vi "运维调试_质控单元.vi"() -> ()   [LabVIEW 2016, in "质控单元.lvlib"]
uses:
  <vilib>/Utility/miscctls.llb/LVPointTypeDef.ctl
  <vilib>/Plasmionique/MB Master/MB_Master_Serial/MB_Master_Serial.lvclass
  F:/Program Files/National Instruments/LabVIEW 2016/vi.lib/Plasmionique/MB Master/MB_Master/MB_Master.lvclass
  <vilib>/Plasmionique/MB Master/MB Master.lvlib
  <vilib>/ptbypt/NI_PtbyPt.lvlib
panel:
  out "COD液位传感器":bool
  out "氨氮总磷液位传感器":bool
  out "columns":string[](array[string])
  out "data":T1
  out "氨氮加标回收测完标志":bool
  out "COD加标回收测完标志":bool
  out "氨氮总磷加标回收测完标志":bool
  out "COD平行样测完标志":bool
  out "氨氮总磷平行样测完标志":bool
  out "输出簇 2":T2
  out "常规启动 2":bool
  out "直接启动 2":bool
  out "启动模块 2":cluster{"氨氮1":bool, "总磷1":bool, " COD1":bool}
  in  "停止测量":bool
  out "输出簇":T2
  in  "启动流程":T3(ring)
  out "启动模块":cluster{"氨氮1":bool, "总磷1":bool, " COD1":bool}
  out "直接启动":bool
  out "常规启动":bool
  out "COD传感器故障报警":bool
  in  "加标回收":bool
  in  "平行样测试":bool
  out "氨氮传感器故障报警":bool
  in  "CODMn停止":bool
  in  "CODMn排液":bool
  in  "CODMn调试":bool
  in  "总磷停止":bool
  in  "总磷排液":bool
  in  "总磷调试":bool
  out "CODMn加标回收率":dbl caption="加标回收率" format="%.2f"
  out "CODMn加标体积":dbl caption="加标体积" format="%.3f"
  out "CODMn母液浓度":dbl caption="加标母液浓度" format="%.2f"
  out "CODMn加标水杯定容体积":dbl caption="加标水杯定容体积" format="%.2f"
  out "CODMn加标后水样浓度":dbl caption="加标后水样浓度" format="%.2f"
  out "CODMn加标前水样浓度":dbl caption="加标前水样浓度" format="%.2f"
  out "CODMn检出限":dbl caption="检出限" format="%.2f"
  out "CODMn量程":dbl caption="量程" format="%.2f"
  out "CODMn状态":u16(ring) caption="状态" items=["待机", "润洗", "进样", "等待取液", "排液"]
  out "总磷加标回收率":dbl caption="加标回收率" format="%.2f"
  out "总磷加标体积":dbl caption="加标体积" format="%.3f"
  out "总磷母液浓度":dbl caption="加标母液浓度" format="%.3f"
  out "总磷加标水杯定容体积":dbl caption="加标水杯定容体积" format="%.2f"
  out "总磷加标后水样浓度":dbl caption="加标后水样浓度" format="%.3f"
  out "总磷加标前水样浓度":dbl caption="加标前水样浓度" format="%.3f"
  out "总磷检出限":dbl caption="检出限" format="%.3f"
  out "总磷量程":dbl caption="量程" format="%.2f"
  out "总磷状态":u16(ring) caption="状态" items=["待机", "润洗", "进样", "等待取液", "排液"]
  out "氨氮加标回收率":dbl caption="加标回收率" format="%.2f"
  out "氨氮加标体积":dbl caption="加标体积" format="%.3f"
  out "氨氮母液浓度":dbl caption="加标母液浓度" format="%.3f"
  out "氨氮加标水杯定容体积":dbl caption="加标水杯定容体积" format="%.2f"
  out "氨氮加标后水样浓度":dbl caption="加标后水样浓度" format="%.3f"
  out "氨氮加标前水样浓度":dbl caption="加标前水样浓度" format="%.3f"
  out "氨氮检出限":dbl caption="检出限" format="%.3f"
  out "氨氮量程":dbl caption="量程" format="%.2f"
  out "氨氮状态":u16(ring) caption="状态" items=["待机", "润洗", "进样", "等待取液", "排液"]
  in  "氨氮停止":bool
  in  "氨氮排液":bool
  in  "氨氮调试":bool
  # "CODMn质控参数"
  # "%"
  # "mL"
  # "mg/L"
  # "mL"
  # "mg/L"
  # "mg/L"
  # "mg/L"
  # "mg/L"
  # "总磷质控参数"
  # "%"
  # "mL"
  # "mg/L"
  # "mL"
  # "mg/L"
  # "mg/L"
  # "mg/L"
  # "mg/L"
  # "氨氮质控参数"
  # "%"
  # "mL"
  # "mg/L"
  # "mL"
  # "mg/L"
  # "mg/L"
  # "mg/L"
  # "mg/L"
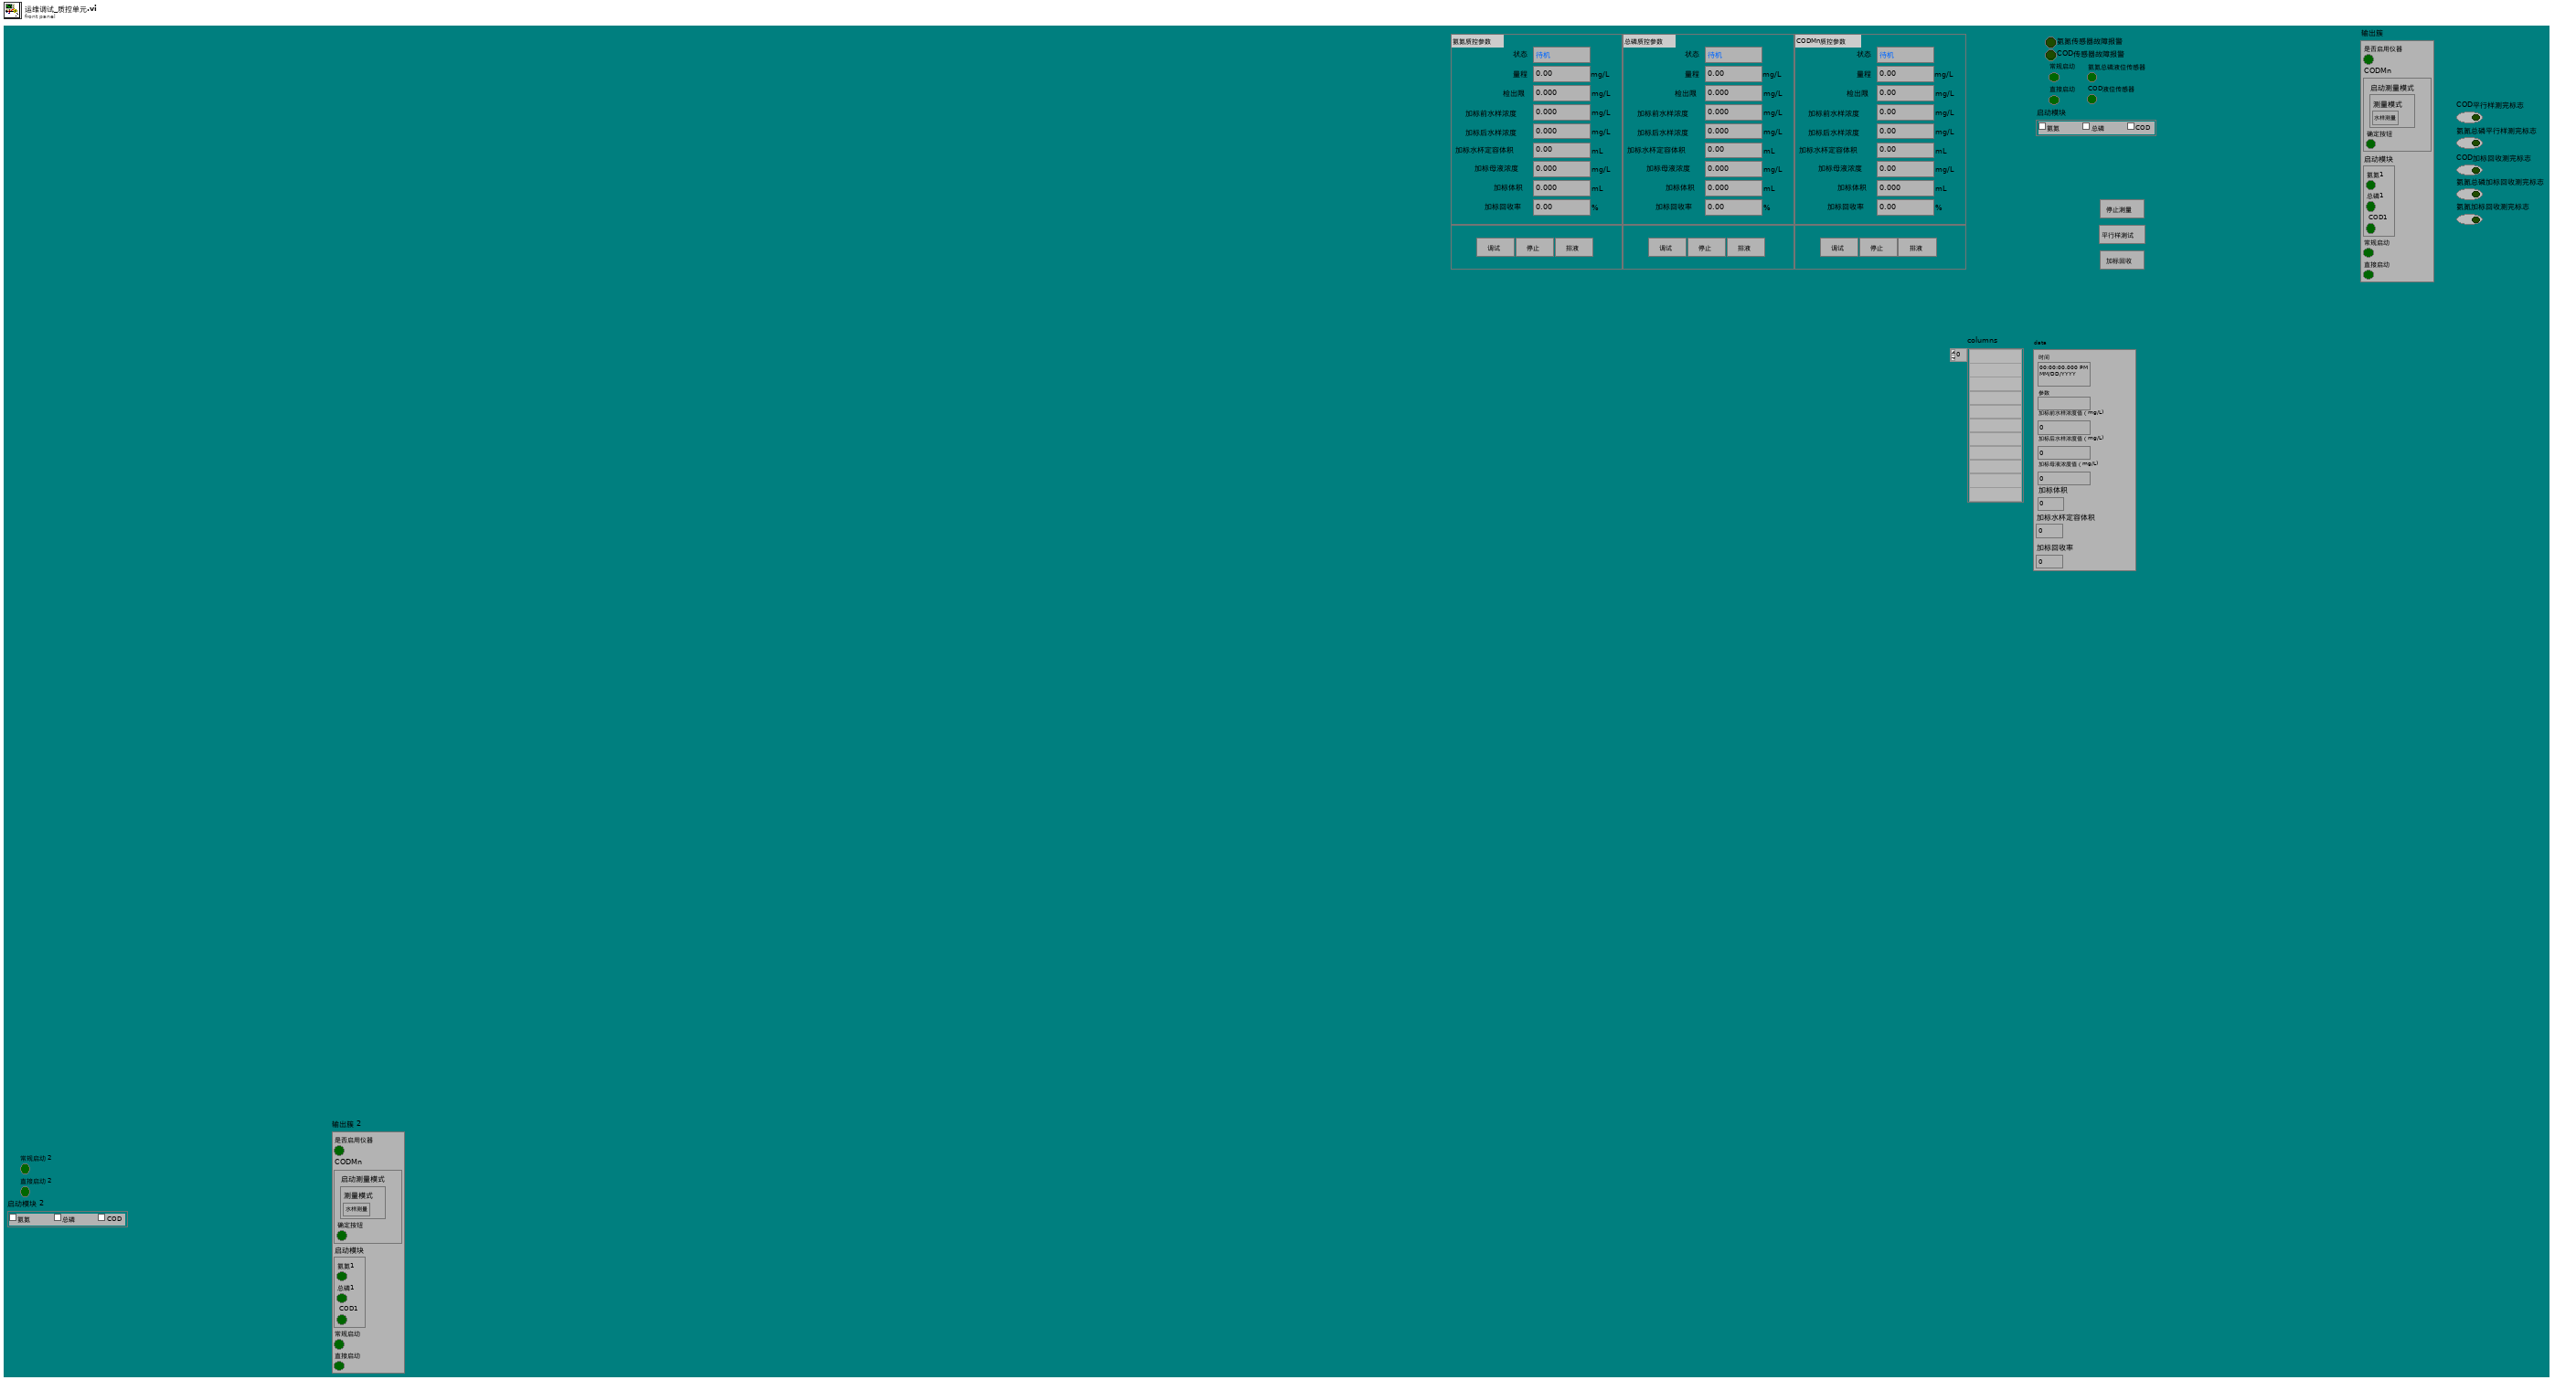
[diagram p1: front panel]
types:
  T1 = cluster{"时间":timestamp, "参数":string, "加标前水样浓度值（mg/L)":sgl, "加标后水样浓度值（mg/L)":sgl, "加标母液浓度值（mg/L)":sgl, "加标体积":dbl, "加标水杯定容体积":dbl, "加标回收率":dbl}
  T2 = cluster{"是否启用仪器":bool, "CODMn":cluster{"启动测量模式":cluster{"测量模式":enum16{"水样测量", "标样核查", "加标回收", "平行样", "校零", "校标"}}, "确定按钮":bool}, "启动模块":cluster{"氨氮1":bool, "总磷1":bool, " COD1":bool}, "常规启动":bool, "直接启动":bool}
  T3 = enum16{"初始化", "采配水", "测量水样", "加标", "取样测量", "测量结束"}
  T4 = cluster{"baud rate (bps)":u32, "stop bits":u16, "parity":u16, "flow control":u16, "timeout":u32, "retries":i32}
  T5 = typedef "LVPointTypeDef.ctl" = cluster{"Horizontal":i16, "Vertical":i16}
  T6 = cluster{"量程":dbl, "检出限":dbl, "加标前水样浓度":dbl, "加标后水样浓度":dbl, "加标水杯定容体积":dbl, "加标母液浓度":dbl, "加标体积":dbl, "加标回收率":dbl}
  T7 = cluster{"因子编码":u32, "单位":u16, "标样参考值":sgl, "水样数据时间":timestamp, "水样实测值":sgl, "水样数据标识":string, "标样数据时间":timestamp, "标样实测值":sgl, "标样数据标识":string, "空白数据时间":timestamp, "空白实测值":sgl, "空白数据标识":string, "零点核查数据时间":timestamp, "零点核查实测值":sgl, "零点核查数据标识":string, "跨度核查数据时间":timestamp, "跨度核查实测值":sgl, "跨度核查数据标识":string, "加标回收数据时间":timestamp, "加标回收实测值":sgl, "加标回收数据标识":string, "平行样数据时间":timestamp, "平行样实测值":sgl, "平行样数据标识":string}
  T8 = cluster{"时间":timestamp, "测量模式":string, "数据类型":string, "检测值":sgl, "单位":string, "数据标识":string, "因子编码":string, "标样参考值":sgl, "ORP-A":sgl, "ORP-B":sgl, "ORP-K":sgl, "COD滴定值":sgl, "高锰酸钾滴定数":sgl, "温度":sgl}
  T9 = enum8{"Enabled", "Disabled", "Disabled and Grayed Out"}
  T10 = cluster{"命令":string, cluster{"starting address":u16, "holding register value":u16}}
  T11 = enum32{"Bad", "Idle", "Run top level", "Running"}
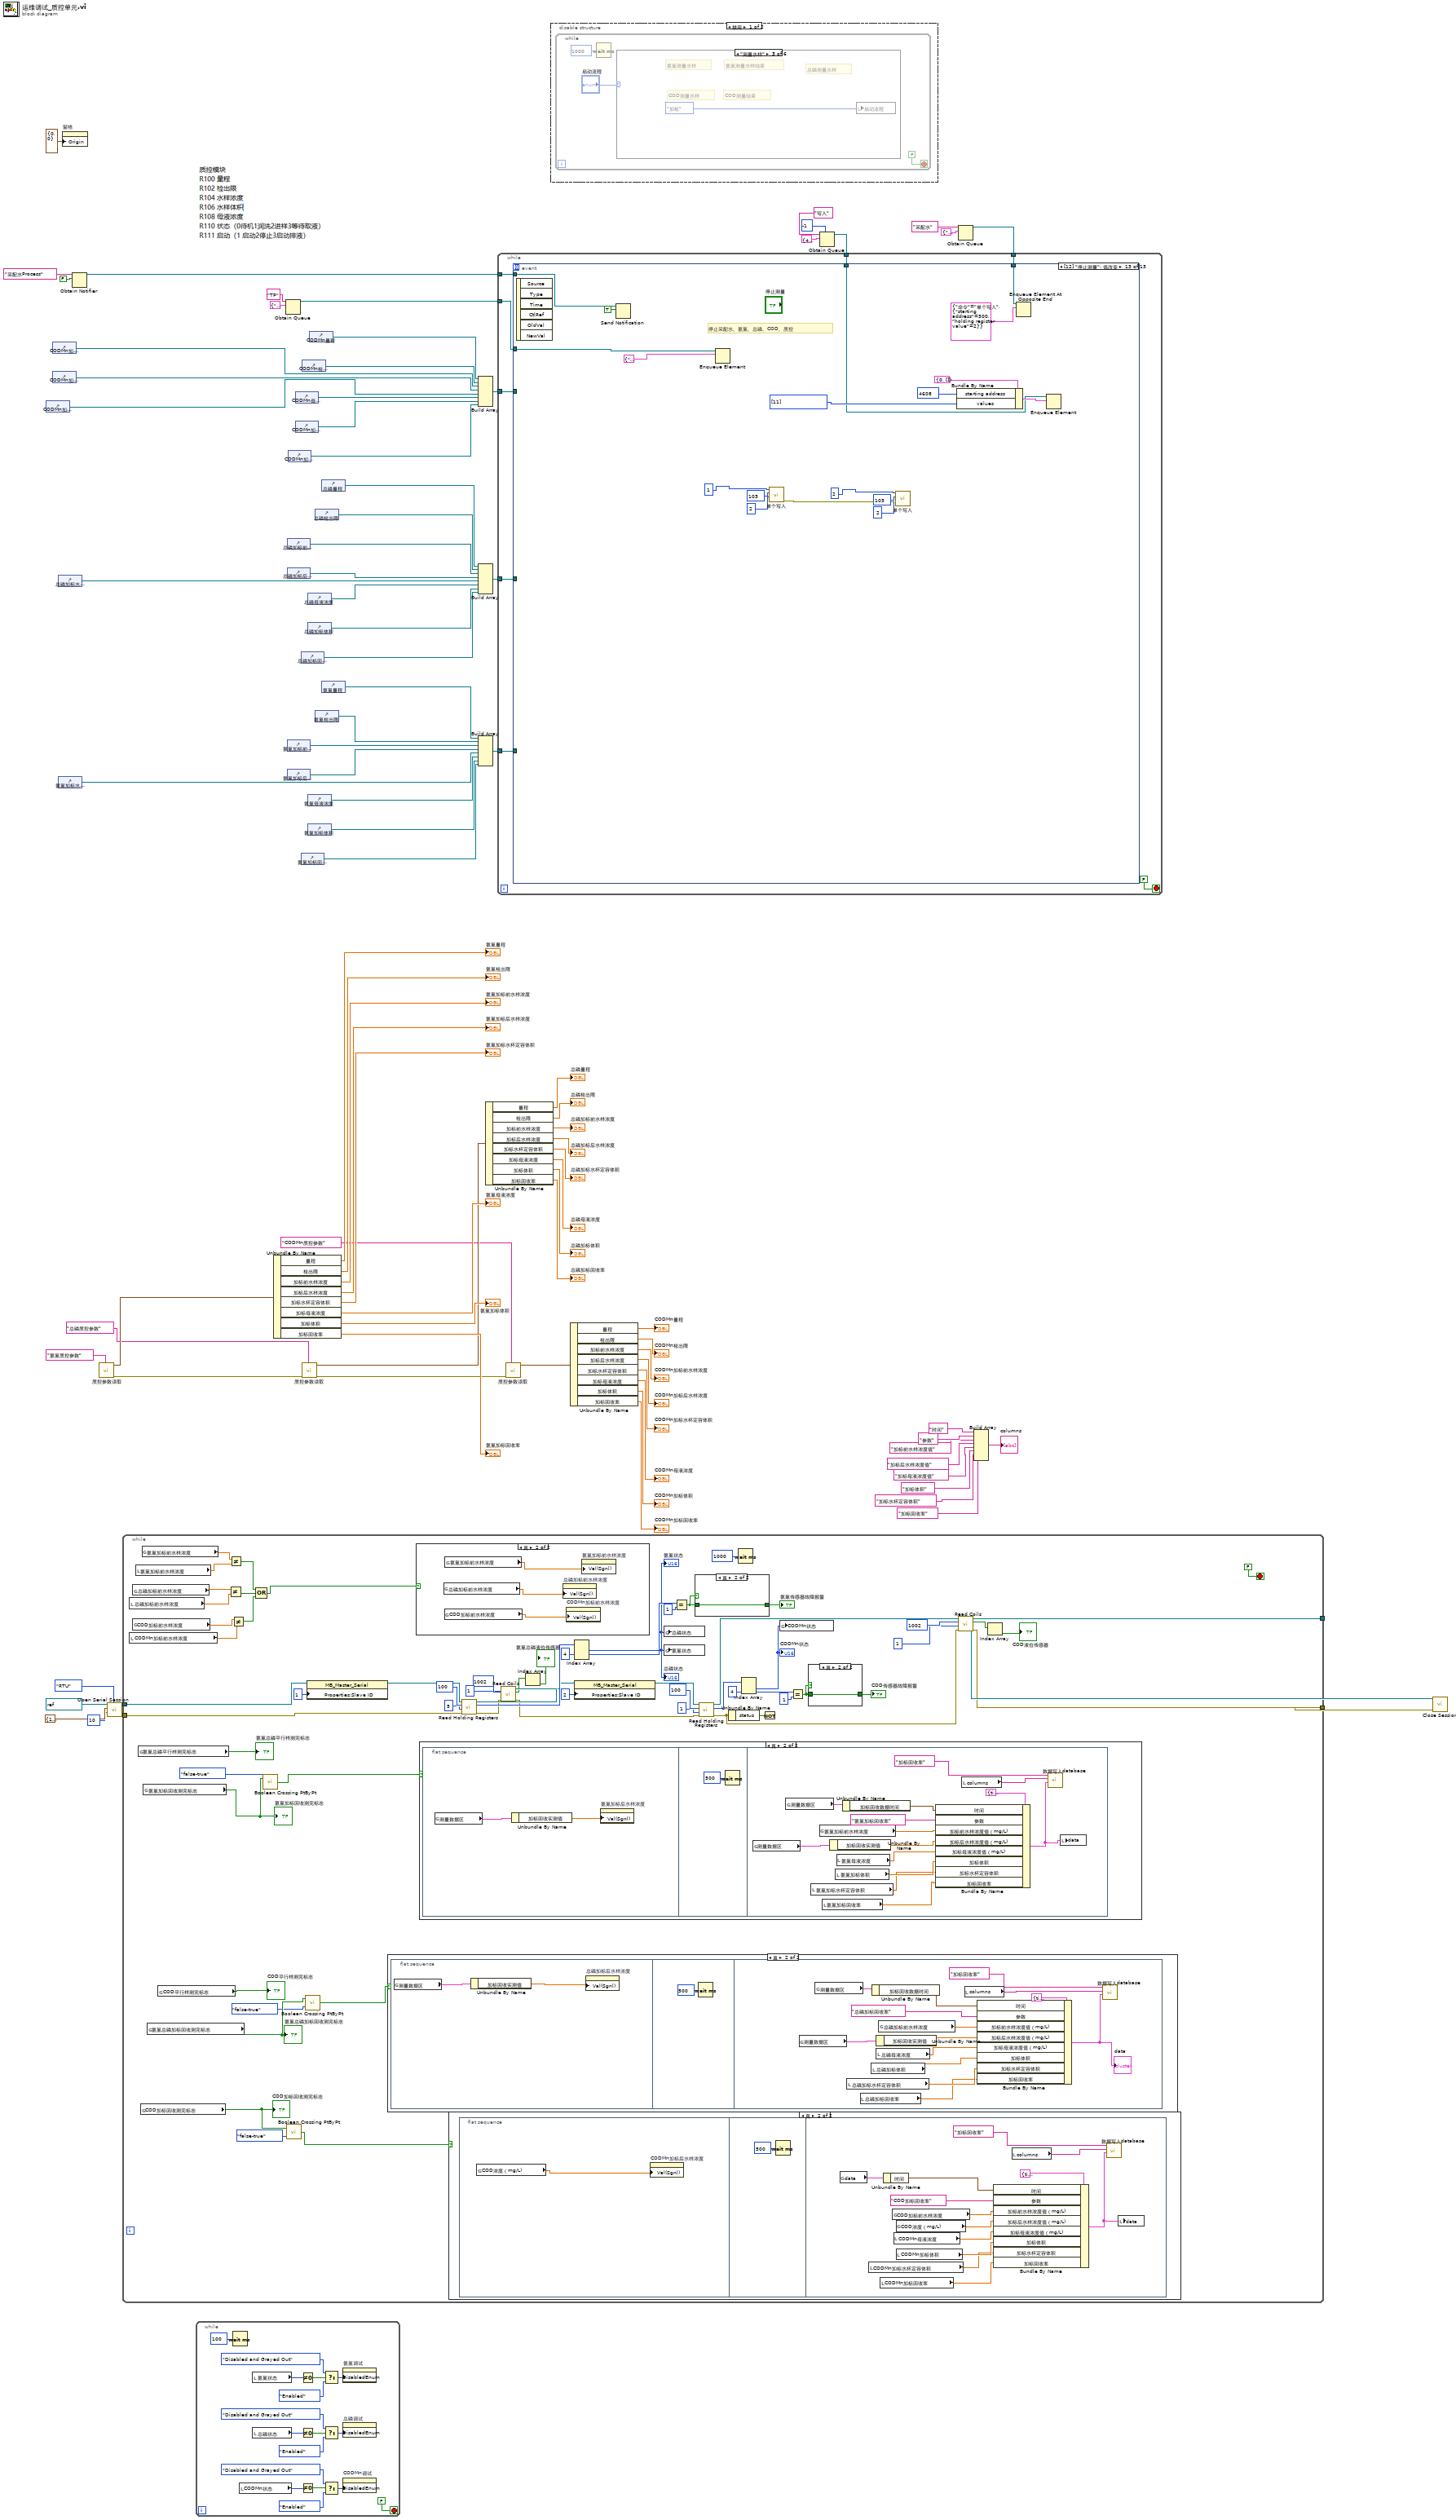
[diagram p0: block diagram]
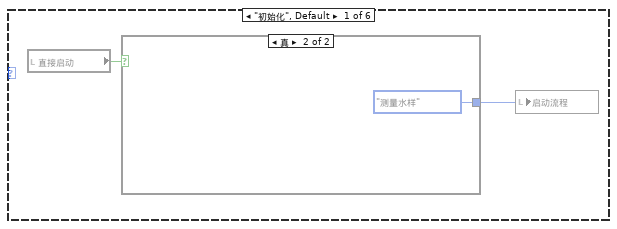
[diagram p2: hidden frame]
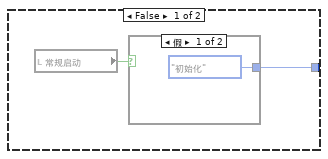
[diagram p3: hidden frame]
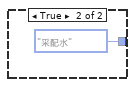
[diagram p4: hidden frame]
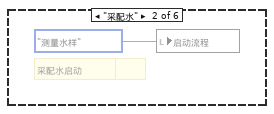
[diagram p5: hidden frame]
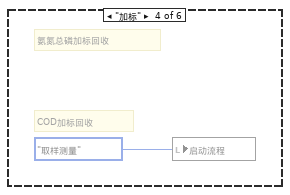
[diagram p6: hidden frame]
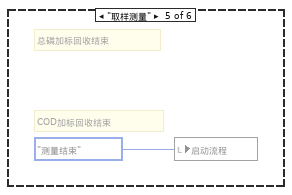
[diagram p7: hidden frame]
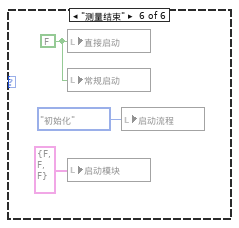
[diagram p8: hidden frame]
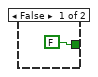
[diagram p14: hidden frame]
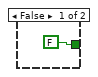
[diagram p15: hidden frame]
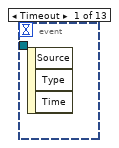
[diagram p16: hidden frame]
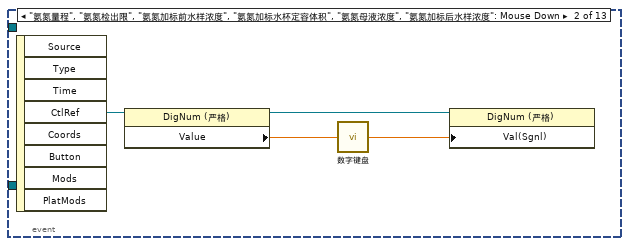
[diagram p17: hidden frame]
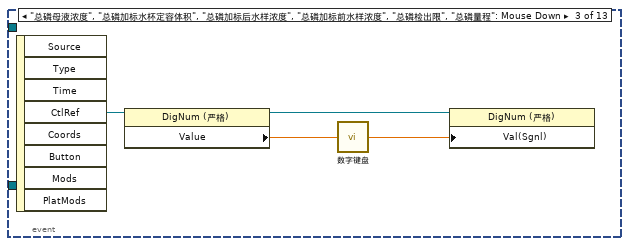
[diagram p18: hidden frame]
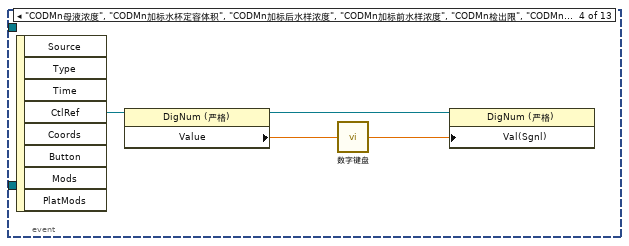
[diagram p19: hidden frame]
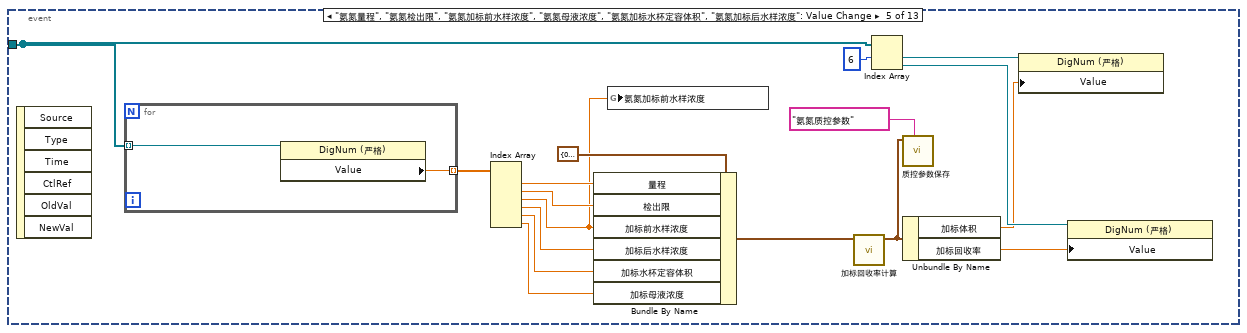
[diagram p20: hidden frame]
diagram:
  n1 = control-ref of="CODMn加标水杯定容体积"() -> (w35:refnum<vi>)
  n2 = control-ref of="CODMn加标前水样浓度"() -> (w37:refnum<vi>)
  n3 = control-ref of="CODMn加标后水样浓度"() -> (w36:refnum<vi>)
  n4 = control-ref of="总磷加标水杯定容体积"() -> (w44:refnum<vi>)
  n5 = control-ref of="氨氮加标水杯定容体积"() -> (w86:refnum<vi>)
  n6 = property on="窗格" class="Pane"("Origin"=T5 {"Horizontal"=0, "Vertical"=0} ("原点")) -> ()  [unwired: 2 in, 2 out]
  n7 = Obtain Notifier(name (unnamed)="采配水Process" ("名称（未命名）"), notification data type=FALSE) -> (notifier out=w20:refnum<notifier>)  [unwired: 2 in, 2 out]
  n8 = call "质控参数读取.vi"("section"="氨氮质控参数") -> ("error out"=w60:errorcluster, "参数"=w79:T6)  [unwired: 9 in]
  n9 = call <vilib>:"Open Serial Session.vi"("Mode (RTU)"=enum16{"RTU", "ASCII"}."RTU", "Slave ID"=u8 10, "Serial Config"=T4 {"baud rate (bps)"=115200, "stop bits"=10, "parity"=0, "flow control"=0, "timeout"=100, "retries"=1}, "VISA Resource"=refnum<visa-resource-name> "COM6") -> ("Error out"=w29:errorcluster, "MB_Serial session"=w30:refnum<class "MB_Master_Serial.lvclass">)  [unwired: 6 in]
  n10 = while {
    tunnel: w30 -> [w152]
    tunnel: w29 -> [w151]
    tunnel: [w97] -> w28
    tunnel: [w91] -> w27
    stop <- FALSE stop-if-true
    n11 = local read "总磷加标前水样浓度"() -> (w122:dbl)
    n12 = local read "CODMn加标前水样浓度"() -> (w120:dbl)
    n13 = global read "水样浓度全局.vi" "COD加标前水样浓度"() -> (w121:dbl)
    n14 = global read "水样浓度全局.vi" "总磷加标前水样浓度"() -> (w123:dbl)
    n15 = local read "氨氮加标前水样浓度"() -> (w124:dbl)
    n16 = global read "质控测完标志全局 1.vi" "氨氮总磷平行样测完标志"() -> (→"氨氮总磷平行样测完标志":bool)
    n17 = global read "质控测完标志全局 1.vi" "COD加标回收测完标志"() -> (w107:bool)
    "COD加标回收测完标志" <- w107
    n18 = global read "水样浓度全局.vi" "氨氮加标前水样浓度"() -> (w125:dbl)
    n19 = global read "质控测完标志全局 1.vi" "氨氮加标回收测完标志"() -> (w113:bool)
    "氨氮加标回收测完标志" <- w113
    n20 = global read "质控测完标志全局 1.vi" "氨氮总磷加标回收测完标志"() -> (w110:bool)
    "氨氮总磷加标回收测完标志" <- w110
    n21 = global read "质控测完标志全局 1.vi" "COD平行样测完标志"() -> (→"COD平行样测完标志":bool)
    n22 = Not Equal?(x=w123, y=w122) -> (x != y?=w117:bool)
    n23 = Not Equal?(x=w125, y=w124) -> (x != y?=w119:bool)
    n24 = Not Equal?(x=w121, y=w120) -> (x != y?=w116:bool)
    n25 = Compound Arithmetic op=OR ("复合运算")(w119, w117, w116) -> (w118:bool)
    n26 = call <vilib>:"Boolean Crossing PtByPt.vi"("direction"=enum16{"either", "false-true", "true-false"}."false-true", "input"=w113) -> ("crossing"=w112:bool)  [unwired: 1 in]
    n27 = call <vilib>:"Boolean Crossing PtByPt.vi"("direction"=enum16{"either", "false-true", "true-false"}."false-true", "input"=w107) -> ("crossing"=w105:bool)  [unwired: 1 in]
    n28 = call <vilib>:"Boolean Crossing PtByPt.vi"("direction"=enum16{"either", "false-true", "true-false"}."false-true", "input"=w110) -> ("crossing"=w108:bool)  [unwired: 1 in]
    n29 = property class="MB_Master_Serial"(reference=w152, "Properties:Slave ID"=u8 1 ("Slave ID")) -> (reference out=w139:refnum<class "MB_Master_Serial.lvclass">)  [unwired: 1 in, 1 out]
    n30 = case shown="真" w108 {
      frame False {
      }
      frame True {
        n31 = flat-sequence {
          frame #0 {
            n32 = global read "VAR总磷氨氮全局变量.vi" "测量数据区"() -> (w171:T7)
            n33 = Unbundle By Name(w171) -> ("加标回收实测值"=w170:sgl)
            n34 = property on="总磷加标后水样浓度" class="DigNum (严格)"("Val(Sgnl)"=w170) -> ()  [unwired: 2 in, 2 out]
          }
          frame #1 {
            n35 = Wait (ms)(milliseconds to wait=u32 500 ("等待时间（毫秒）")) -> ()  [unwired: 1 out]
          }
          frame #2 {
            n36 = global read "VAR总磷氨氮全局变量.vi" "测量数据区"() -> (w181:T7)
            n37 = global read "VAR总磷氨氮全局变量.vi" "测量数据区"() -> (w174:T7)
            n38 = local read "总磷加标水杯定容体积"() -> (w177:dbl)
            n39 = local read "总磷加标回收率"() -> (w176:dbl)
            n40 = local read "总磷加标体积"() -> (w178:dbl)
            n41 = Unbundle By Name(w174) -> ("加标回收数据时间"=w173:timestamp)
            n42 = Unbundle By Name(w181) -> ("加标回收实测值"=w180:sgl)
            n43 = local read "总磷母液浓度"() -> (w179:dbl)
            n44 = global read "水样浓度全局.vi" "总磷加标前水样浓度"() -> (w182:dbl)
            n45 = local read "columns"() -> (w185:string[])
            n46 = Bundle By Name(cluster=T1 {"时间"=timestamp(0 s since 1904-01-01), "参数"="", "加标前水样浓度值（mg/L)"=0.0, "加标后水样浓度值（mg/L)"=0.0, "加标母液浓度值（mg/L)"=0.0, "加标体积"=0.0, "加标水杯定容体积"=0.0, "加标回收率"=0.0} ("data"), "时间"=w173, "参数"="总磷加标回收率" ("table"), "加标前水样浓度值（mg/L)"=w182, "加标后水样浓度值（mg/L)"=w180, "加标母液浓度值（mg/L)"=w179, "加标体积"=w178, "加标水杯定容体积"=w177, "加标回收率"=w176) -> (w175:T1)
            "data" <- w175
            n47 = call "数据写入database.vi"("data"=w175, "columns"=w185, "table"="加标回收率") -> ()  [unwired: 9 in]
          }
        }
      }
    }
    n48 = case shown="真" w118 {
      frame False {
      }
      frame True {
        n49 = global read "水样浓度全局.vi" "总磷加标前水样浓度"() -> (w205:dbl)
        n50 = global read "水样浓度全局.vi" "COD加标前水样浓度"() -> (w204:dbl)
        n51 = global read "水样浓度全局.vi" "氨氮加标前水样浓度"() -> (w206:dbl)
        n52 = property on="总磷加标前水样浓度" class="DigNum (严格)"("Val(Sgnl)"=w205) -> ()  [unwired: 2 in, 2 out]
        n53 = property on="CODMn加标前水样浓度" class="DigNum (严格)"("Val(Sgnl)"=w204) -> ()  [unwired: 2 in, 2 out]
        n54 = property on="氨氮加标前水样浓度" class="DigNum (严格)"("Val(Sgnl)"=w206) -> ()  [unwired: 2 in, 2 out]
      }
    }
    n55 = case shown="真" w112 {
      frame False {
      }
      frame True {
        n56 = flat-sequence {
          frame #0 {
            n57 = global read "VAR总磷氨氮全局变量.vi" "测量数据区"() -> (w188:T7)
            n58 = Unbundle By Name(w188) -> ("加标回收实测值"=w187:sgl)
            n59 = property on="氨氮加标后水样浓度" class="DigNum (严格)"("Val(Sgnl)"=w187) -> ()  [unwired: 2 in, 2 out]
          }
          frame #1 {
            n60 = Wait (ms)(milliseconds to wait=u32 500 ("等待时间（毫秒）")) -> ()  [unwired: 1 out]
          }
          frame #2 {
            n61 = global read "VAR总磷氨氮全局变量.vi" "测量数据区"() -> (w196:T7)
            n62 = global read "VAR总磷氨氮全局变量.vi" "测量数据区"() -> (w200:T7)
            n63 = local read "氨氮加标水杯定容体积"() -> (w192:dbl)
            n64 = global read "水样浓度全局.vi" "氨氮加标前水样浓度"() -> (w197:dbl)
            n65 = local read "氨氮加标回收率"() -> (w191:dbl)
            n66 = Unbundle By Name(w196) -> ("加标回收实测值"=w195:sgl)
            n67 = local read "氨氮加标体积"() -> (w193:dbl)
            n68 = local read "氨氮母液浓度"() -> (w194:dbl)
            n69 = Unbundle By Name(w200) -> ("加标回收数据时间"=w199:timestamp)
            n70 = Bundle By Name(cluster=T1 {"时间"=timestamp(0 s since 1904-01-01), "参数"="", "加标前水样浓度值（mg/L)"=0.0, "加标后水样浓度值（mg/L)"=0.0, "加标母液浓度值（mg/L)"=0.0, "加标体积"=0.0, "加标水杯定容体积"=0.0, "加标回收率"=0.0} ("data"), "时间"=w199, "参数"="氨氮加标回收率" ("table"), "加标前水样浓度值（mg/L)"=w197, "加标后水样浓度值（mg/L)"=w195, "加标母液浓度值（mg/L)"=w194, "加标体积"=w193, "加标水杯定容体积"=w192, "加标回收率"=w191) -> (w190:T1)
            n71 = local read "columns"() -> (w202:string[])
            n72 = call "数据写入database.vi"("data"=w190, "columns"=w202, "table"="加标回收率") -> ()  [unwired: 9 in]
            n73 = local write "data"(w190) -> ()
          }
        }
      }
    }
    n74 = case shown="真" w105 {
      frame False {
      }
      frame True {
        n75 = flat-sequence {
          frame #0 {
            n76 = global read "COD浓度全局变量.vi" "COD浓度（mg/L)"() -> (w155:dbl)
            n77 = property on="CODMn加标后水样浓度" class="DigNum (严格)"("Val(Sgnl)"=w155) -> ()  [unwired: 2 in, 2 out]
          }
          frame #1 {
            n78 = Wait (ms)(milliseconds to wait=u32 500 ("等待时间（毫秒）")) -> ()  [unwired: 1 out]
          }
          frame #2 {
            n79 = global read "COD读取DATA全局.vi" "data"() -> (w165:T8)
            n80 = local read "CODMn加标水杯定容体积"() -> (w159:dbl)
            n81 = local read "CODMn加标回收率"() -> (w158:dbl)
            n82 = Unbundle By Name(w165) -> ("时间"=w164:timestamp)
            n83 = global read "水样浓度全局.vi" "COD加标前水样浓度"() -> (w163:dbl)
            n84 = local read "CODMn母液浓度"() -> (w161:dbl)
            n85 = global read "COD浓度全局变量.vi" "COD浓度（mg/L)"() -> (w162:dbl)
            n86 = local read "CODMn加标体积"() -> (w160:dbl)
            n87 = Bundle By Name(cluster=T1 {"时间"=timestamp(0 s since 1904-01-01), "参数"="", "加标前水样浓度值（mg/L)"=0.0, "加标后水样浓度值（mg/L)"=0.0, "加标母液浓度值（mg/L)"=0.0, "加标体积"=0.0, "加标水杯定容体积"=0.0, "加标回收率"=0.0} ("data"), "时间"=w164, "参数"="COD加标回收率" ("table"), "加标前水样浓度值（mg/L)"=w163, "加标后水样浓度值（mg/L)"=w162, "加标母液浓度值（mg/L)"=w161, "加标体积"=w160, "加标水杯定容体积"=w159, "加标回收率"=w158) -> (w157:T1)
            n88 = local read "columns"() -> (w168:string[])
            n89 = call "数据写入database.vi"("data"=w157, "columns"=w168, "table"="加标回收率") -> ()  [unwired: 9 in]
            n90 = local write "data"(w157) -> ()
          }
        }
      }
    }
    n91 = call <vilib>:"Read Holding Registers.vi"("error in (no error)"=w151, "quantity"=u16 5, "starting address"=u16 100, "MB session in"=w139) -> ("error out"=w100:errorcluster, "Registers"=w147:u16[], "MB session out"=w142:refnum<class "MB_Master_Serial.lvclass">)  [unwired: 5 in]
    n92 = call <vilib>:"Read Coils.vi"("error in (no error)"=w100, "quantity"=u16 1, "starting address"=u16 1002, "MB session in"=w142) -> ("error out"=w99:errorcluster, "Coils"=w101:bool[], "MB session out"=w104:refnum<class "MB_Master_Serial.lvclass">)  [unwired: 5 in]
    n93 = Index Array(array=w101) -> (element=→"氨氮总磷液位传感器":bool)  [unwired: 1 in]
    n94 = Index Array(array=w147, index #2=4 ("索引")) -> (element #1=w127:u16, element #2=w136:u16)  [unwired: 2 in, 1 out]
    "氨氮状态" <- w127
    "总磷状态" <- w127
    n95 = property class="MB_Master_Serial"(reference=w104, "Properties:Slave ID"=u8 2 ("Slave ID")) -> (reference out=w141:refnum<class "MB_Master_Serial.lvclass">)  [unwired: 1 in, 1 out]
    n96 = global write "氨氮加标回收状态全局变量.vi" "总磷状态"(w127) -> ()
    n97 = global write "氨氮加标回收状态全局变量.vi" "氨氮状态"(w127) -> ()
    n98 = Equal?(x=w136, y=u16 1) -> (x = y?=w133:bool)
    n99 = case shown="真" w133 {
      tunnel: w133 -> [_ w210]
      tunnel: [FALSE w210] -> w134
      frame False {
      }
      frame True {
      }
    }
    "氨氮传感器故障报警" <- w134
    n100 = call <vilib>:"Read Holding Registers.vi"("error in (no error)"=w99, "quantity"=u16 1, "starting address"=u16 100, "MB session in"=w141) -> ("error out"=w92:errorcluster, "Registers"=w146:u16[], "MB session out"=w150:refnum<class "MB_Master_Serial.lvclass">)  [unwired: 5 in]
    n101 = Unbundle By Name(w92) -> ("status"=w143:bool)
    n102 = Wait (ms)(milliseconds to wait=u32 1000 ("等待时间（毫秒）")) -> ()  [unwired: 1 out]
    n103 = Index Array(array=w146, index #2=4 ("索引")) -> (element #1=w126:u16, element #2=w130:u16)  [unwired: 1 in]
    "CODMn状态" <- w126
    n104 = Not(x=w143) -> ()  [unwired: 1 out]
    n105 = global write "氨氮加标回收状态全局变量.vi" "CODMn状态"(w126) -> ()
    n106 = Equal?(x=w130, y=u16 1) -> (x = y?=w128:bool)
    n107 = case shown="真" w128 {
      tunnel: w128 -> [_ w208]
      tunnel: [FALSE w208] -> w129
      frame False {
      }
      frame True {
      }
    }
    "COD传感器故障报警" <- w129
    n108 = call <vilib>:"Read Coils.vi"("error in (no error)"=w92, "quantity"=u16 1, "starting address"=u16 1002, "MB session in"=w150) -> ("error out"=w91:errorcluster, "Coils"=w94:bool[], "MB session out"=w97:refnum<class "MB_Master_Serial.lvclass">)  [unwired: 5 in]
    n109 = Index Array(array=w94) -> (element=→"COD液位传感器":bool)  [unwired: 1 in]
  }
  n110 = while {
    stop <- FALSE stop-if-true
    n111 = Wait (ms)(milliseconds to wait=u32 100 ("等待时间（毫秒）")) -> ()  [unwired: 1 out]
    n112 = local read "CODMn状态"() -> (w212:u16)
    n113 = local read "氨氮状态"() -> (w226:u16)
    n114 = local read "总磷状态"() -> (w217:u16)
    n115 = Not Equal To 0?(x=w226) -> (x != 0?=w225:bool)
    n116 = Not Equal To 0?(x=w217) -> (x != 0?=w219:bool)
    n117 = Not Equal To 0?(x=w212) -> (x != 0?=w216:bool)
    n118 = Select(t=T9."Disabled and Grayed Out" ("禁用"), s=w225, f=T9."Enabled") -> (s? t:f=w222:T9)
    n119 = Select(t=T9."Disabled and Grayed Out" ("禁用"), s=w219, f=T9."Enabled") -> (s? t:f=w218:T9)
    n120 = Select(t=T9."Disabled and Grayed Out" ("禁用"), s=w216, f=T9."Enabled") -> (s? t:f=w213:T9)
    n121 = property on="氨氮调试" class="Bool"("DisabledEnum"=w222) -> ()  [unwired: 2 in, 2 out]
    n122 = property on="总磷调试" class="Bool"("DisabledEnum"=w218) -> ()  [unwired: 2 in, 2 out]
    n123 = property on="CODMn调试" class="Bool"("DisabledEnum"=w213) -> ()  [unwired: 2 in, 2 out]
  }
  n124 = Unbundle By Name(w79) -> ("量程"=→"氨氮量程":dbl, "检出限"=→"氨氮检出限":dbl, "加标前水样浓度"=→"氨氮加标前水样浓度":dbl, "加标后水样浓度"=→"氨氮加标后水样浓度":dbl, "加标水杯定容体积"=→"氨氮加标水杯定容体积":dbl, "加标母液浓度"=→"氨氮母液浓度":dbl, "加标体积"=→"氨氮加标体积":dbl, "加标回收率"=→"氨氮加标回收率":dbl)
  n125 = Obtain Queue(name (unnamed)="TP" ("名称（未命名）"), element data type=cluster{"命令":string, "data":variant} {"命令"="", "data"=variant}) -> (queue out=w8:refnum<queue>)  [unwired: 3 in, 2 out]
  n126 = control-ref of="总磷加标前水样浓度"() -> (w46:refnum<vi>)
  n127 = control-ref of="总磷加标后水样浓度"() -> (w45:refnum<vi>)
  n128 = control-ref of="氨氮加标前水样浓度"() -> (w87:refnum<vi>)
  n129 = control-ref of="氨氮加标后水样浓度"() -> (w83:refnum<vi>)
  n130 = control-ref of="CODMn加标回收率"() -> (w32:refnum<vi>)
  n131 = control-ref of="CODMn母液浓度"() -> (w34:refnum<vi>)
  n132 = control-ref of="CODMn加标体积"() -> (w33:refnum<vi>)
  n133 = control-ref of="总磷加标回收率"() -> (w42:refnum<vi>)
  n134 = control-ref of="氨氮加标回收率"() -> (w81:refnum<vi>)
  n135 = control-ref of="CODMn检出限"() -> (w38:refnum<vi>)
  n136 = call "质控参数读取.vi"("section"="总磷质控参数", "error in (no error)"=w60) -> ("error out"=w57:errorcluster, "参数"=w69:T6)  [unwired: 8 in]
  n137 = control-ref of="总磷母液浓度"() -> (w43:refnum<vi>)
  n138 = control-ref of="总磷加标体积"() -> (w41:refnum<vi>)
  n139 = control-ref of="氨氮母液浓度"() -> (w85:refnum<vi>)
  n140 = control-ref of="氨氮加标体积"() -> (w82:refnum<vi>)
  n141 = control-ref of="CODMn量程"() -> (w39:refnum<vi>)
  n142 = control-ref of="总磷检出限"() -> (w47:refnum<vi>)
  n143 = control-ref of="氨氮检出限"() -> (w88:refnum<vi>)
  n144 = control-ref of="总磷量程"() -> (w48:refnum<vi>)
  n145 = control-ref of="氨氮量程"() -> (w89:refnum<vi>)
  n146 = Build Array(w39, w38, w37, w36, w35, w34, w33, w32) -> (w31:refnum<vi>[])
  n147 = Build Array(w48, w47, w46, w45, w44, w43, w41, w42) -> (w40:refnum<vi>[])
  n148 = Build Array(w89, w88, w87, w83, w86, w85, w82, w81) -> (w84:refnum<vi>[])
  n149 = Unbundle By Name(w69) -> ("量程"=→"总磷量程":dbl, "检出限"=→"总磷检出限":dbl, "加标前水样浓度"=→"总磷加标前水样浓度":dbl, "加标后水样浓度"=→"总磷加标后水样浓度":dbl, "加标水杯定容体积"=→"总磷加标水杯定容体积":dbl, "加标母液浓度"=→"总磷母液浓度":dbl, "加标体积"=→"总磷加标体积":dbl, "加标回收率"=→"总磷加标回收率":dbl)
  n150 = call "质控参数读取.vi"("section"="CODMn质控参数", "error in (no error)"=w57) -> ("参数"=w59:T6)  [unwired: 8 in, 1 out]
  n151 = disable-structure shown="禁用" {
    frame Disabled {
      n152 = while {
        stop <- FALSE stop-if-true
        n153 = Wait (ms)(milliseconds to wait=u32 1000 ("等待时间（毫秒）")) -> ()  [unwired: 1 out]
        n154 = case shown="\"测量水样\"" "启动流程" {
          frame "初始化", Default {
            n155 = local read "直接启动"() -> (w232:bool)
            n156 = case shown="真" w232 {
              tunnel: [w233 T3."测量水样" ("启动流程")] -> w231
              frame False {
                n157 = local read "常规启动"() -> (w234:bool)
                n158 = case shown="假" w234 {
                  tunnel: [T3."初始化" ("启动流程") T3."采配水" ("启动流程")] -> w233
                  frame False {
                  }
                  frame True {
                  }
                }
              }
              frame True {
              }
            }
            n159 = local write "启动流程"(w231) -> ()
          }
          frame "采配水" {
            # "采配水启动结束"
            # "采配水启动"
            n160 = local write "启动流程"(T3."测量水样" ("启动流程")) -> ()
          }
          frame "测量水样" {
            # "总磷测量水样"
            # "COD测量结束"
            # "总磷测量结束"
            # "氨氮测量水样结束"
            # "COD测量水样"
            # "氨氮测量水样"
            n161 = local write "启动流程"(T3."加标" ("启动流程")) -> ()
          }
          frame "加标" {
            # "COD加标回收"
            # "氨氮总磷加标回收"
            n162 = local write "启动流程"(T3."取样测量" ("启动流程")) -> ()
          }
          frame "取样测量" {
            # "COD加标回收结束"
            # "总磷加标回收结束"
            n163 = local write "启动流程"(T3."测量结束" ("启动流程")) -> ()
          }
          frame "测量结束" {
            w243 = FALSE ("直接启动")
            n164 = local write "直接启动"(w243) -> ()
            n165 = local write "常规启动"(w243) -> ()
            n166 = local write "启动模块"(cluster{"氨氮1":bool, "总磷1":bool, " COD1":bool} {"氨氮1"=FALSE, "总磷1"=FALSE, " COD1"=FALSE} ("启动模块")) -> ()
            n167 = local write "启动流程"(T3."初始化" ("启动流程")) -> ()
          }
        }
      }
    }
    frame Enabled {
    }
  }
  n168 = Unbundle By Name(w59) -> ("量程"=→"CODMn量程":dbl, "检出限"=→"CODMn检出限":dbl, "加标前水样浓度"=→"CODMn加标前水样浓度":dbl, "加标后水样浓度"=→"CODMn加标后水样浓度":dbl, "加标水杯定容体积"=→"CODMn加标水杯定容体积":dbl, "加标母液浓度"=→"CODMn母液浓度":dbl, "加标体积"=→"CODMn加标体积":dbl, "加标回收率"=→"CODMn加标回收率":dbl)
  n169 = Obtain Queue(max queue size (-1, unlimited)=-1 ("队列最大值（-1，无限）"), name (unnamed)="写入" ("名称（未命名）"), element data type=cluster{"starting address":u16, "values":u16[]} {"starting address"=4272, "values"=[]}) -> (queue out=w4:refnum<queue>)  [unwired: 2 in, 2 out]
  n170 = Obtain Queue(name (unnamed)="采配水" ("名称（未命名）"), element data type=cluster{"命令":string, "数据":variant} {"命令"="", "数据"=variant}) -> (queue out=w1:refnum<queue>)  [unwired: 3 in, 2 out]
  n171 = while {
    tunnel: w84 -> [w251]
    tunnel: w40 -> [w250]
    tunnel: w31 -> [w249]
    tunnel: w20 -> [w248]
    tunnel: w8 -> [w247]
    tunnel: w4 -> [w246]
    tunnel: w1 -> [w245]
    stop <- FALSE stop-if-true
    n172 = event shown="[12] \"停止测量\": 值改变" {
      selector: _ -> [_ _ _ _ _ _ _ _ _ _ _ _ _]
      dyn-events: _ -> [_ _ _ _ _ _ _ _ _ _ _ _ _]
      timeout: _ -> [_ _ _ _ _ _ _ _ _ _ _ _ _]
      tunnel: w251 -> [_ _ _ _ w271 _ _ w328 _ _ _ _ _]
      tunnel: w250 -> [_ _ _ _ _ w285 _ w325 _ _ _ _ _]
      tunnel: w249 -> [_ _ _ _ _ _ w304 w324 _ _ _ _ _]
      tunnel: w248 -> [_ _ _ _ _ _ _ _ _ _ w349 w375 w417]
      tunnel: w247 -> [_ _ _ _ _ _ _ _ _ _ _ _ w414]
      tunnel: w246 -> [_ _ _ _ _ _ _ _ _ _ _ _ w409]
      tunnel: w245 -> [_ _ _ _ _ _ _ _ _ _ _ _ w400]
      event Timeout {
        n173 = event-data() -> ()  [unwired: 1 in, 3 out]
      }
      event "氨氮量程", "氨氮检出限", "氨氮加标前水样浓度", "氨氮加标水杯定容体积", "氨氮母液浓度", "氨氮加标后水样浓度": Mouse Down {
        n174 = event-data() -> ("CtlRef"=w256:refnum<vi>)  [unwired: 1 in, 7 out]
        n175 = property class="DigNum (严格)"(reference=w256) -> (reference out=w254:refnum<vi>, "Value"=w255:dbl)  [unwired: 1 in, 1 out]
        n176 = call "数字键盘.vi"("OldNumber"=w255) -> ("NewNumber"=w253:sgl)
        n177 = property class="DigNum (严格)"(reference=w254, "Val(Sgnl)"=w253) -> ()  [unwired: 1 in, 2 out]
      }
      event "总磷母液浓度", "总磷加标水杯定容体积", "总磷加标后水样浓度", "总磷加标前水样浓度", "总磷检出限", "总磷量程": Mouse Down {
        n178 = event-data() -> ("CtlRef"=w260:refnum<vi>)  [unwired: 1 in, 7 out]
        n179 = property class="DigNum (严格)"(reference=w260) -> (reference out=w258:refnum<vi>, "Value"=w259:dbl)  [unwired: 1 in, 1 out]
        n180 = call "数字键盘.vi"("OldNumber"=w259) -> ("NewNumber"=w257:sgl)
        n181 = property class="DigNum (严格)"(reference=w258, "Val(Sgnl)"=w257) -> ()  [unwired: 1 in, 2 out]
      }
      event "CODMn母液浓度", "CODMn加标水杯定容体积", "CODMn加标后水样浓度", "CODMn加标前水样浓度", "CODMn检出限", "CODMn量程": Mouse Down {
        n182 = event-data() -> ("CtlRef"=w264:refnum<vi>)  [unwired: 1 in, 7 out]
        n183 = property class="DigNum (严格)"(reference=w264) -> (reference out=w262:refnum<vi>, "Value"=w263:dbl)  [unwired: 1 in, 1 out]
        n184 = call "数字键盘.vi"("OldNumber"=w263) -> ("NewNumber"=w261:sgl)
        n185 = property class="DigNum (严格)"(reference=w262, "Val(Sgnl)"=w261) -> ()  [unwired: 1 in, 2 out]
      }
      event "氨氮量程", "氨氮检出限", "氨氮加标前水样浓度", "氨氮母液浓度", "氨氮加标水杯定容体积", "氨氮加标后水样浓度": Value Change {
        n186 = event-data() -> ()  [unwired: 1 in, 6 out]
        n187 = for {
          tunnel: w271 -> [w283] mode=indexing
          tunnel: [w282] -> w280 mode=indexing
          n188 = property class="DigNum (严格)"(reference=w283) -> ("Value"=w282:dbl)  [unwired: 1 in, 2 out]
        }
        n189 = Index Array(array=w280) -> (element #1=w279:dbl, element #2=w278:dbl, element #3=w265:dbl, element #4=w277:dbl, element #5=w276:dbl, element #6=w274:dbl)  [unwired: 6 in]
        n190 = Bundle By Name(cluster=T6 {"量程"=0.0, "检出限"=0.0, "加标前水样浓度"=0.0, "加标后水样浓度"=0.0, "加标水杯定容体积"=0.0, "加标母液浓度"=0.0, "加标体积"=0.0, "加标回收率"=0.0} ("参数"), "量程"=w279, "检出限"=w278, "加标前水样浓度"=w265, "加标后水样浓度"=w277, "加标水杯定容体积"=w276, "加标母液浓度"=w274) -> (w273:T6)
        n191 = global write "水样浓度全局.vi" "氨氮加标前水样浓度"(w265) -> ()
        n192 = call "加标回收率计算.vi"("参数"=w273) -> ("参数 out"=w272:T6)  [unwired: 10 in]
        n193 = Index Array(array=w271, index #1=6 ("索引")) -> (element #1=w270:refnum<vi>, element #2=w268:refnum<vi>)  [unwired: 1 in]
        n194 = call "质控参数保存.vi"("section"="氨氮质控参数", "参数"=w272) -> ()  [unwired: 9 in, 1 out]
        n195 = Unbundle By Name(w272) -> ("加标体积"=w266:dbl, "加标回收率"=w267:dbl)
        n196 = property class="DigNum (严格)"(reference=w270, "Value"=w266) -> ()  [unwired: 1 in, 2 out]
        n197 = property class="DigNum (严格)"(reference=w268, "Value"=w267) -> ()  [unwired: 1 in, 2 out]
      }
      event "总磷母液浓度", "总磷加标水杯定容体积", "总磷加标后水样浓度", "总磷加标前水样浓度", "总磷检出限", "总磷量程": Value Change {
        n198 = event-data() -> ()  [unwired: 1 in, 6 out]
        n199 = for {
          tunnel: w285 -> [w302] mode=indexing
          tunnel: [w301] -> w299 mode=indexing
          n200 = property class="DigNum (严格)"(reference=w302) -> ("Value"=w301:dbl)  [unwired: 1 in, 2 out]
        }
        n201 = Index Array(array=w299) -> (element #1=w298:dbl, element #2=w297:dbl, element #3=w284:dbl, element #4=w296:dbl, element #5=w295:dbl, element #6=w293:dbl)  [unwired: 6 in]
        n202 = global write "水样浓度全局.vi" "总磷加标前水样浓度"(w284) -> ()
        n203 = Bundle By Name(cluster=T6 {"量程"=0.0, "检出限"=0.0, "加标前水样浓度"=0.0, "加标后水样浓度"=0.0, "加标水杯定容体积"=0.0, "加标母液浓度"=0.0, "加标体积"=0.0, "加标回收率"=0.0} ("参数"), "量程"=w298, "检出限"=w297, "加标前水样浓度"=w284, "加标后水样浓度"=w296, "加标水杯定容体积"=w295, "加标母液浓度"=w293) -> (w292:T6)
        n204 = call "加标回收率计算.vi"("参数"=w292) -> ("参数 out"=w291:T6)  [unwired: 10 in]
        n205 = Index Array(array=w285, index #1=6 ("索引")) -> (element #1=w290:refnum<vi>, element #2=w287:refnum<vi>)  [unwired: 1 in]
        n206 = call "质控参数保存.vi"("section"="总磷质控参数", "参数"=w291) -> ()  [unwired: 9 in, 1 out]
        n207 = Unbundle By Name(w291) -> ("加标体积"=w288:dbl, "加标回收率"=w286:dbl)
        n208 = property class="DigNum (严格)"(reference=w290, "Value"=w288) -> ()  [unwired: 1 in, 2 out]
        n209 = property class="DigNum (严格)"(reference=w287, "Value"=w286) -> ()  [unwired: 1 in, 2 out]
      }
      event "CODMn母液浓度", "CODMn加标水杯定容体积", "CODMn加标后水样浓度", "CODMn加标前水样浓度", "CODMn检出限", "CODMn量程": Value Change {
        n210 = event-data() -> ()  [unwired: 1 in, 6 out]
        n211 = for {
          tunnel: w304 -> [w321] mode=indexing
          tunnel: [w320] -> w318 mode=indexing
          n212 = property class="DigNum (严格)"(reference=w321) -> ("Value"=w320:dbl)  [unwired: 1 in, 2 out]
        }
        n213 = Index Array(array=w318) -> (element #1=w317:dbl, element #2=w316:dbl, element #3=w303:dbl, element #4=w315:dbl, element #5=w314:dbl, element #6=w312:dbl)  [unwired: 6 in]
        n214 = global write "水样浓度全局.vi" "COD加标前水样浓度"(w303) -> ()
        n215 = Bundle By Name(cluster=T6 {"量程"=0.0, "检出限"=0.0, "加标前水样浓度"=0.0, "加标后水样浓度"=0.0, "加标水杯定容体积"=0.0, "加标母液浓度"=0.0, "加标体积"=0.0, "加标回收率"=0.0} ("参数"), "量程"=w317, "检出限"=w316, "加标前水样浓度"=w303, "加标后水样浓度"=w315, "加标水杯定容体积"=w314, "加标母液浓度"=w312) -> (w311:T6)
        n216 = call "加标回收率计算.vi"("参数"=w311) -> ("参数 out"=w310:T6)  [unwired: 10 in]
        n217 = Index Array(array=w304, index #1=6 ("索引")) -> (element #1=w309:refnum<vi>, element #2=w306:refnum<vi>)  [unwired: 1 in]
        n218 = call "质控参数保存.vi"("section"="CODMn质控参数", "参数"=w310) -> ()  [unwired: 9 in, 1 out]
        n219 = Unbundle By Name(w310) -> ("加标体积"=w307:dbl, "加标回收率"=w305:dbl)
        n220 = property class="DigNum (严格)"(reference=w309, "Value"=w307) -> ()  [unwired: 1 in, 2 out]
        n221 = property class="DigNum (严格)"(reference=w306, "Value"=w305) -> ()  [unwired: 1 in, 2 out]
      }
      event "氨氮调试", "总磷调试", "CODMn调试": Value Change {
        n222 = event-data() -> ("CtlRef"=w327:refnum<vi>)  [unwired: 1 in, 5 out]
        n223 = property class="Bool"(reference=w327) -> ("Label.Text"=w326:string)  [unwired: 1 in, 2 out]
        n224 = case shown="\"总磷调试\"" w326 {
          tunnel: w328 -> [w329 _ _]
          tunnel: w325 -> [_ w331 _]
          tunnel: w324 -> [_ _ w333]
          tunnel: ["氨氮模块" ("标题") "总磷模块" ("标题") "CODMn模块" ("标题")] -> w323
          tunnel: [w329 w331 w333] -> w322
          frame "氨氮调试", Default {
          }
          frame "总磷调试" {
          }
          frame "CODMn调试" {
          }
        }
        n225 = call "加标模块单控对话框.vi"("数组"=w322, "标题"=w323) -> ()  [unwired: 10 in]
      }
      event "氨氮停止", "总磷停止", "CODMn停止": Value Change {
        n226 = event-data() -> ("CtlRef"=w339:refnum<vi>)  [unwired: 1 in, 5 out]
        n227 = property class="Bool"(reference=w339) -> ("Label.Text"=w338:string)  [unwired: 1 in, 2 out]
        n228 = case shown="\"氨氮停止\", \"总磷停止\", 默认" w338 {
          tunnel: [u8 1 ("Slave ID") u8 2 ("Slave ID")] -> w335
          frame "氨氮停止", "总磷停止", Default {
          }
          frame "CODMn停止" {
          }
        }
        n229 = call "单个写入.vi"("value"=u16 2, "address"=u16 103, "Slave ID"=w335) -> ()  [unwired: 8 in, 1 out]
      }
      event "氨氮排液", "CODMn排液", "总磷排液": Value Change {
        n230 = event-data() -> ("CtlRef"=w346:refnum<vi>)  [unwired: 1 in, 5 out]
        n231 = property class="Bool"(reference=w346) -> ("Label.Text"=w345:string)  [unwired: 1 in, 2 out]
        n232 = case shown="\"氨氮排液\", \"总磷排液\", 默认" w345 {
          tunnel: [u8 1 ("Slave ID") u8 2 ("Slave ID")] -> w342
          frame "氨氮排液", "总磷排液", Default {
          }
          frame "CODMn排液" {
          }
        }
        n233 = call "单个写入.vi"("value"=u16 3, "address"=u16 103, "Slave ID"=w342) -> ()  [unwired: 8 in, 1 out]
      }
      event "加标回收": Value Change {
        n234 = event-data() -> ()  [unwired: 1 in, 6 out]
        n235 = flat-sequence {
          tunnel: [w357] -> w352
          tunnel: [w356] -> w351
          tunnel: [w355] -> w350
          tunnel: w349 -> [w353]
          tunnel: w352 -> [w364]
          tunnel: w351 -> [w363]
          tunnel: w350 -> [w362]
          frame #0 {
            n236 = Send Notification(notification=FALSE ("通知"), notifier=w353) -> ()  [unwired: 1 in, 2 out]
            n237 = call "质控启动流程对话框.vi"() -> ("启动模块"=w357:cluster{"氨氮1":bool, "总磷1":bool, " COD1":bool}, "直接启动"=w355:bool, "常规启动"=w356:bool)  [unwired: 8 in, 1 out]
            "常规启动" <- w356
            "直接启动" <- w355
            "启动模块" <- w357
          }
          frame #1 {
            n238 = Bundle By Name(cluster=T2 {"是否启用仪器"=FALSE, "CODMn"={"启动测量模式"={"测量模式"=enum."水样测量"}, "确定按钮"=TRUE}, "启动模块"={"氨氮1"=FALSE, "总磷1"=FALSE, " COD1"=FALSE}, "常规启动"=FALSE, "直接启动"=FALSE} ("参数"), "是否启用仪器"=TRUE, "启动模块"=w364, "常规启动"=w363, "直接启动"=w362) -> (w359:T2)
            "输出簇" <- w359
            n239 = vi-ref "古田户外一体站流程质控自动启动.vi"() -> (w360:refnum<vi>)
            n240 = property class="VI"(reference=w360) -> ("Name"=w361:string, "Exec.State"=w358:T11)  [unwired: 1 in, 2 out]
            n241 = case shown="\"Idle\"" w358 {
              tunnel: w361 -> [_ w372]
              tunnel: w359 -> [_ w371]
              frame "Bad", Default {
              }
              frame "Idle" {
                n242 = Open VI Reference(type specifier VI Refnum (for type only)=refnum<vi> refnum ("类型说明符VI引用句柄（仅用于类型）"), vi path=w372, options=128 ("选项")) -> (vi reference=w374:refnum<vi>, error out=w368:errorcluster)  [unwired: 3 in]
                n243 = call-by-ref "开始异步调用"(reference=w374, error in=w368, "参数"=w371) -> (reference out=w370:refnum<vi>, error out=w369:errorcluster)  [unwired: 11 in]
                n244 = Close Reference(reference=w370, error in (no error)=w369) -> ()  [unwired: 1 out]
              }
            }
          }
        }
      }
      event "平行样测试": Value Change {
        n245 = event-data() -> ()  [unwired: 1 in, 6 out]
        n246 = flat-sequence {
          tunnel: [w380] -> w378
          tunnel: [w382] -> w377
          tunnel: [w381] -> w376
          tunnel: w375 -> [w379]
          tunnel: w378 -> [w389]
          tunnel: w377 -> [w388]
          tunnel: w376 -> [w387]
          frame #0 {
            n247 = Cancel Notification(0:w379) -> ()  [unwired: 1 in, 3 out]
            n248 = call "平行样启动流程对话框.vi"() -> ("启动模块"=w380:cluster{"氨氮1":bool, "总磷1":bool, " COD1":bool}, "直接启动"=w381:bool, "常规启动"=w382:bool)  [unwired: 8 in, 1 out]
            "常规启动 2" <- w382
            "直接启动 2" <- w381
            "启动模块 2" <- w380
          }
          frame #1 {
            n249 = Bundle By Name(cluster=T2 {"是否启用仪器"=FALSE, "CODMn"={"启动测量模式"={"测量模式"=enum."水样测量"}, "确定按钮"=TRUE}, "启动模块"={"氨氮1"=FALSE, "总磷1"=FALSE, " COD1"=FALSE}, "常规启动"=FALSE, "直接启动"=FALSE} ("参数"), "是否启用仪器"=TRUE, "启动模块"=w389, "常规启动"=w388, "直接启动"=w387) -> (w384:T2)
            "输出簇 2" <- w384
            n250 = vi-ref "古田户外一体站流程平行样自动启动.vi"() -> (w385:refnum<vi>)
            n251 = property class="VI"(reference=w385) -> ("Name"=w386:string, "Exec.State"=w383:T11)  [unwired: 1 in, 2 out]
            n252 = case shown="\"Idle\"" w383 {
              tunnel: w386 -> [_ w398]
              tunnel: w384 -> [_ w392]
              frame "Bad", Default {
              }
              frame "Idle" {
                n253 = Open VI Reference(type specifier VI Refnum (for type only)=refnum<vi> refnum ("类型说明符VI引用句柄（仅用于类型）"), vi path=w398, options=128 ("选项")) -> (vi reference=w399:refnum<vi>, error out=w397:errorcluster)  [unwired: 3 in]
                n254 = call-by-ref "开始异步调用"(reference=w399, error in=w397, "参数"=w392) -> (reference out=w394:refnum<vi>, error out=w393:errorcluster)  [unwired: 9 in]
                n255 = Close Reference(reference=w394, error in (no error)=w393) -> ()  [unwired: 1 out]
              }
            }
          }
        }
      }
      event "停止测量": Value Change {
        # "停止采配水、氨氮、总磷、COD、质控"
        n256 = event-data() -> ()  [unwired: 1 in, 6 out]
        n257 = Send Notification(notification=TRUE ("通知"), notifier=w417) -> ()  [unwired: 1 in, 2 out]
        n258 = Enqueue Element(queue=w414, element=cluster{"命令":string, "data":variant} {"命令"="启动", "data"=variant(cluster{"站号":u16, "控制命令输出":u16[]} {"站号"=1, "控制命令输出"=[2816]})} ("元素")) -> ()  [unwired: 2 in, 3 out]
        n259 = call "单个写入.vi"("value"=u16 2, "address"=u16 103, "Slave ID"=u8 1) -> ("error out"=w402:errorcluster)  [unwired: 8 in]
        n260 = call "单个写入.vi"("Error in"=w402, "value"=u16 2, "address"=u16 103, "Slave ID"=u8 2) -> ()  [unwired: 7 in, 1 out]
        n261 = Bundle By Name(cluster=cluster{"starting address":u16, "values":u16[]} {"starting address"=0, "values"=[]}, "starting address"=u16 4608, "values"=u16[] [11]) -> (w411:cluster{"starting address":u16, "values":u16[]})
        n262 = Enqueue Element At Opposite End(queue=w400, element=T10 {"命令"="单个写入", {"starting address"=300, "holding register value"=2}} ("元素")) -> ()  [unwired: 2 in, 3 out]
        n263 = Enqueue Element(queue=w409, element=w411) -> ()  [unwired: 2 in, 3 out]
      }
    }
  }
  n264 = Build Array("时间" ("table"), "参数" ("table"), "加标前水样浓度值" ("元素"), "加标后水样浓度值" ("元素"), "加标母液浓度值" ("元素"), "加标体积" ("元素"), "加标水杯定容体积" ("元素"), "加标回收率" ("元素")) -> (→"columns":string[])
  n265 = call-dynamic "Close Session.vi"("error in (no error)"=w27, "MB_Serial session"=w28) -> ()  [unwired: 9 in, 1 out]
